vi "PD500 - Local Sense Test TSFTS2.vi"(5 "HMP4040 Channel Settings":T2={"CH1 Voltage"=24.0, "CH1 Current"=1.0, "CH1 Output"=TRUE, "CH2 Voltage"=24.0, "CH2 Current"=1.0, "CH2 Output"=TRUE, "CH3 Voltage"=24.0, "CH3 Current"=1.0, "CH3 Output"=TRUE, "CH4 Voltage"=24.0, "CH4 Current"=1.0, "CH4 Output"=TRUE, "Master Output"=TRUE} {"CH4 Current" format="%.3f"; "CH4 Voltage" format="%.3f"; "CH3 Current" format="%.3f"; "CH3 Voltage" format="%.3f"; "CH2 Current" format="%.3f"; "CH2 Voltage" format="%.3f"; "CH1 Current" format="%.3f"; "CH1 Voltage" format="%.3f"}, 10 "Message IN":string, 11 "Board Selector":T1) -> (0 "error out":errorcluster, 1 "Pass?":bool, 2 "Message OUT":string)   [LabVIEW 2022 SP3]
uses:
  HMP4000 Communication/HMP4040_ChannelControl.ctl
  Serial Board Com/Board Select.ctl
panel:
  out "error out 2":errorcluster
  in  "error in (no error) 2":errorcluster
  out "MSE Array":dbl[](array[numeric])
  out "Voltage Readings":dbl[][](array[numeric])
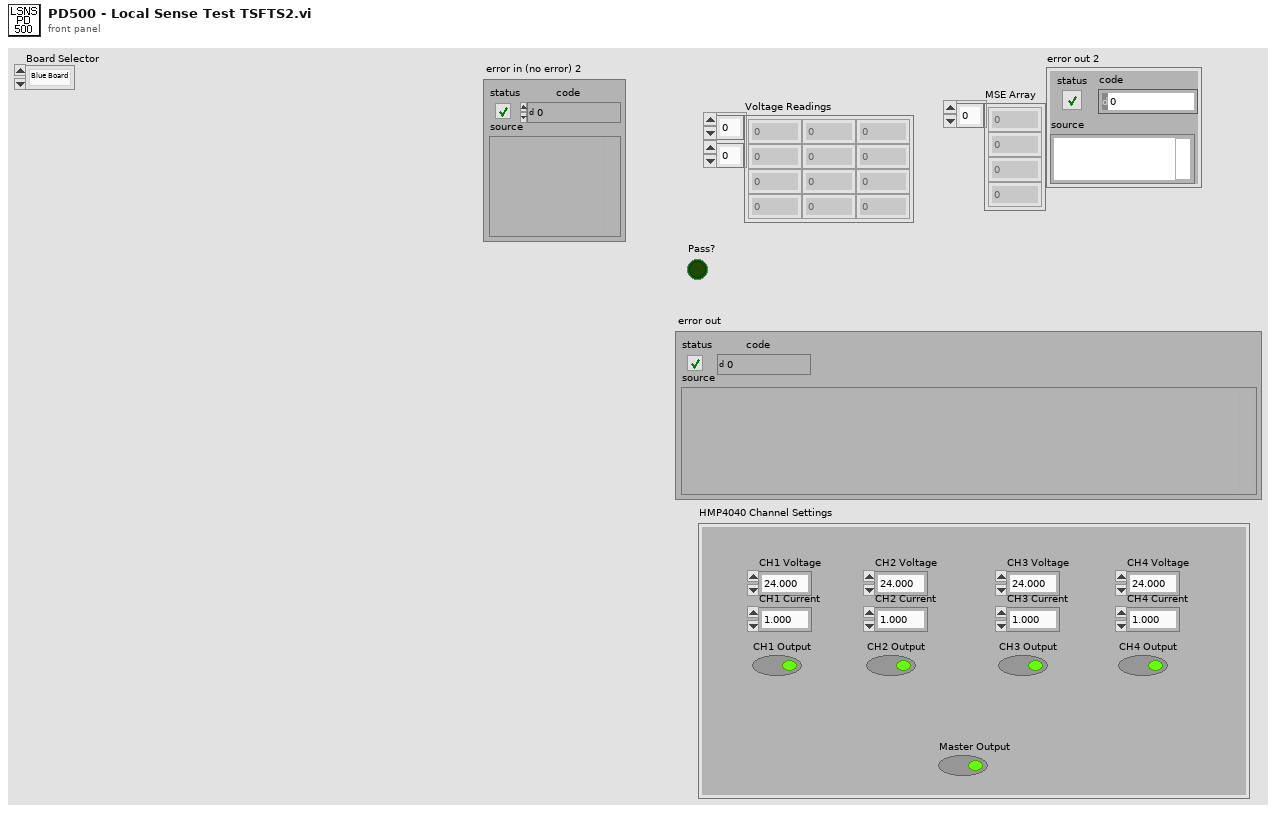
[diagram p1: front panel]
types:
  T1 = typedef "Board Select.ctl" = enum16{"Blue Board", "Green Board"}
  T2 = typedef "HMP4040_ChannelControl.ctl" = cluster{"CH1 Voltage":dbl, "CH1 Current":dbl, "CH1 Output":bool, "CH2 Voltage":dbl, "CH2 Current":dbl, "CH2 Output":bool, "CH3 Voltage":dbl, "CH3 Current":dbl, "CH3 Output":bool, "CH4 Voltage":dbl, "CH4 Current":dbl, "CH4 Output":bool, "Master Output":bool}
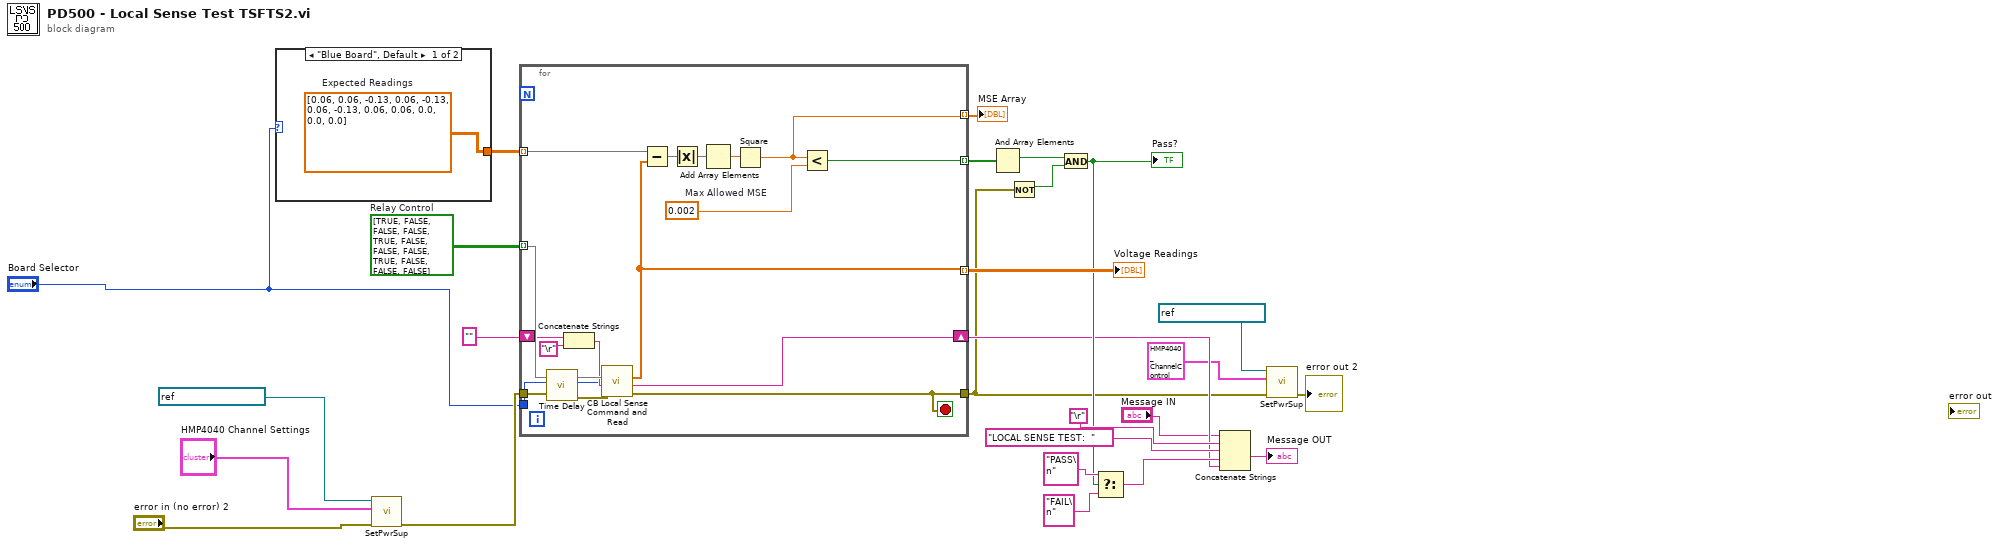
[diagram p0: block diagram]
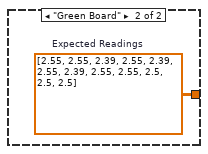
[diagram p2: hidden frame]
diagram:
  w24 = bool[][] [[TRUE, FALSE, FALSE], [FALSE, TRUE, FALSE], [FALSE, FALSE, TRUE], [FALSE, FALSE, FALSE]]  # Relay Control
  n1 = case shown="\"Blue Board\", Default" "Board Selector" {
    tunnel: [w27 w28] -> w26
    frame "Blue Board", Default {
      w27 = dbl[][] [[0.06, 0.06, -0.13], [0.06, -0.13, 0.06], [-0.13, 0.06, 0.06], [0.0, 0.0, 0.0]]  # Expected Readings
    }
    frame "Green Board" {
      w28 = dbl[][] [[2.55, 2.55, 2.39], [2.55, 2.39, 2.55], [2.39, 2.55, 2.55], [2.5, 2.5, 2.5]]  # Expected Readings
    }
  }
  n2 = call "SetPwrSup.vi"("error in (no error)"="error in (no error) 2", "HMP4040 Channel Settings"="HMP4040 Channel Settings", "HMP4040 IN"=refnum<visa-resource-name> "HMP4040_FTS2" ("VISA resource name")) -> ("error out"=w6:errorcluster)  [unwired: 7 in, 1 out]
  n3 = for {
    tunnel: [w45] -> w4
    tunnel: w6 -> [w31]
    tunnel: w26 -> [w42] mode=indexing
    tunnel: [w39] -> w25 mode=indexing
    tunnel: w24 -> [w38] mode=indexing
    tunnel: [w37] -> w21 mode=indexing
    tunnel: [w36] -> w20 mode=indexing
    shift-right: [w35] -> w13
    shift-left: "" -> [w34]
    tunnel: "Board Selector" -> [w29]
    stop <- w45 stop-if-true
    w40 = 0.002  # Max Allowed MSE
    n4 = call "Time Delay"("error in (no error)"=w31) -> ("error out"=w30:errorcluster)  [unwired: 10 in]
    n5 = Concatenate Strings(w34, "\r") -> (w33:string)
    n6 = call "CB Local Sense Command and Read.vi"("Board Selector"=w29, "error in (no error)"=w30, "Message IN"=w33, "Relay Control"=w38) -> ("error out"=w45:errorcluster, "Message OUT"=w35:string, "Voltage Array"=w37:dbl[])  [unwired: 4 in, 1 out]
    n7 = Subtract(x=w42, y=w37) -> (x-y=w44:dbl[])
    n8 = Absolute Value(x=w44) -> (abs(x)=w43:dbl[])
    n9 = Add Array Elements(numeric array=w43) -> (sum=w41:dbl)
    n10 = Square(x=w41) -> (x^2=w36:dbl)
    n11 = Less?(x=w36, y=w40) -> (x < y?=w39:bool)
  }
  "Voltage Readings" <- w21
  "MSE Array" <- w20
  n12 = And Array Elements(Boolean array=w25) -> (logical AND=w23:bool)
  n13 = Not(x=w4) -> (.not. x?=w22:bool)
  n14 = And(x=w23, y=w22) -> (x .and. y?=w15:bool)
  "Pass?" <- w15
  n15 = Select(t="PASS\n", s=w15, f="FAIL\n") -> (s? t:f=w14:string)
  n16 = Concatenate Strings("Message IN", "\r", "LOCAL SENSE TEST:  ", w14, w13) -> (→"Message OUT":string)
  n17 = call "SetPwrSup.vi"("error in (no error)"=w4, "HMP4040 Channel Settings"=T2 {"CH1 Voltage"=24.0, "CH1 Current"=1.0, "CH1 Output"=TRUE, "CH2 Voltage"=24.0, "CH2 Current"=5.0, "CH2 Output"=TRUE, "CH3 Voltage"=24.0, "CH3 Current"=1.0, "CH3 Output"=FALSE, "CH4 Voltage"=24.0, "CH4 Current"=1.0, "CH4 Output"=FALSE, "Master Output"=TRUE}, "HMP4040 IN"=refnum<visa-resource-name> "HMP4040_FTS2" ("VISA resource name")) -> ("error out"=→"error out 2":errorcluster)  [unwired: 7 in, 1 out]
